vi "Data.vi"(11 "Panel Create Msg in":refnum<class "Panel Create Msg.lvclass">) -> (2 "Panel":refnum<class "Helper Loop.lvclass">)   [LabVIEW 2021, in "Panel Create.lvlib" / "Panel Create Msg.lvclass"]
uses:
  Panel Create Msg.lvclass
  Helper Loop/Helper Loop.lvclass
  Panel Create Msg.lvclass/Panel Create Msg.ctl
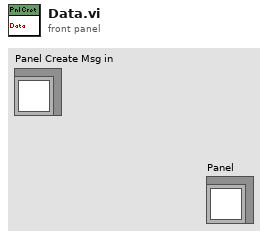
[diagram p1: front panel]
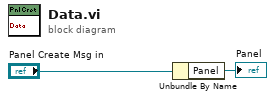
[diagram p0: block diagram]
diagram:
  n1 = Unbundle By Name("Panel Create Msg in") -> ("Panel"=→"Panel":refnum<class "Helper Loop.lvclass">)
